vi "Add if Valid.vi"(10 "element":cluster{"Heat":i32, "Prev Steps":T1[]}, 11 "set in":set{cluster{"Heat":i32, "Prev Steps":T1[]}}(c389)) -> (3 "set out":set{cluster{"Heat":i32, "Prev Steps":T1[]}}(c389))   [LabVIEW 2021, in "Heat Map.lvclass"]
uses:
  Heat Map.lvclass
  Direction.ctl
  Heat Map.lvclass/Heat Map.ctl
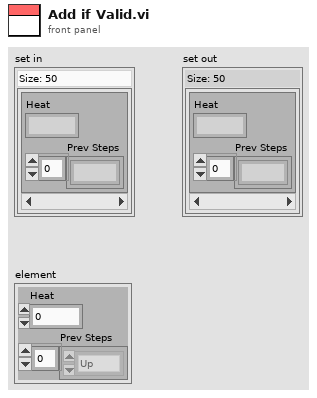
[diagram p1: front panel]
types:
  T1 = typedef "Heat Map.lvclass/Direction.ctl" = enum16{"Up", "Down", "Right", "Left"}
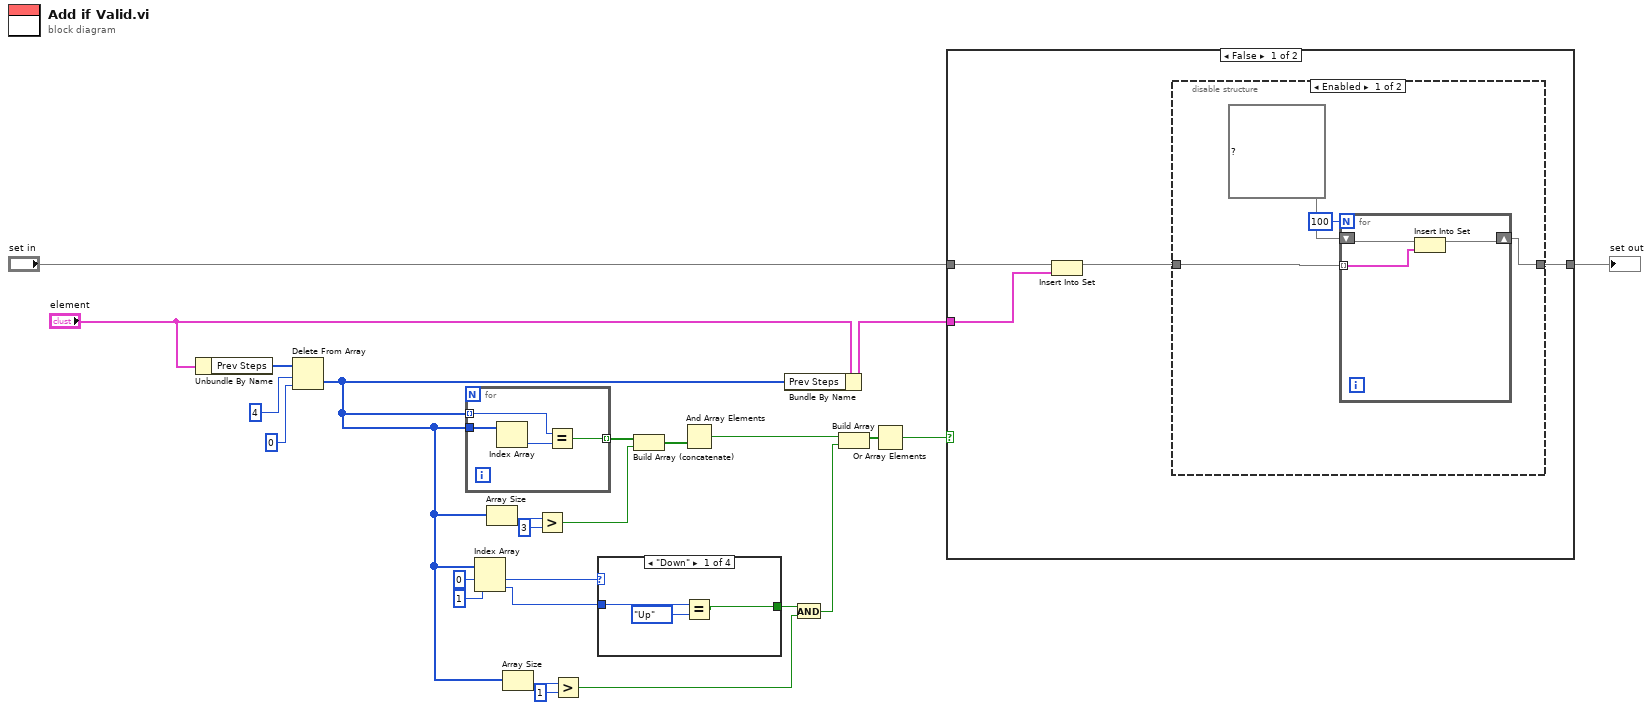
[diagram p0: block diagram]
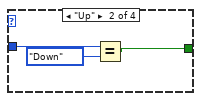
[diagram p4: hidden frame]
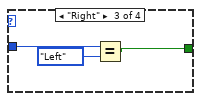
[diagram p5: hidden frame]
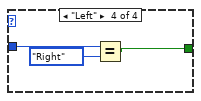
[diagram p6: hidden frame]
diagram:
  n1 = Unbundle By Name("element") -> ("Prev Steps"=w7:T1[])
  n2 = Delete From Array(array=w7, length=4, index=0) -> (deleted portion=w2:T1[])  [unwired: 1 out]
  n3 = for {
    tunnel: w2 -> [w27] mode=indexing
    tunnel: w2 -> [w29]
    tunnel: [w26] -> w23 mode=indexing
    n4 = Index Array(array=w29) -> (element=w28:T1)  [unwired: 1 in]
    n5 = Equal?(x=w27, y=w28) -> (x = y?=w26:bool)
  }
  n6 = Index Array(array=w2, index #1=0 ("index"), index #2=1 ("index")) -> (element #1=w20:T1, element #2=w19:T1)
  n7 = Array Size(array=w2) -> (size(s)=w13:i32)
  n8 = Array Size(array=w2) -> (size(s)=w8:i32)
  n9 = Greater?(x=w13, y=3) -> (0:w11:bool)
  n10 = Greater?(x=w8, y=1) -> (0:w5:bool)
  n11 = case shown="\"Down\"" w20 {
    tunnel: w19 -> [w32 w35 w38 w41]
    tunnel: [w30 w33 w36 w39] -> w17
    frame "Down" {
      n12 = Equal?(x=w32, y=Direction."Up") -> (x = y?=w30:bool)
    }
    frame "Up" {
      n13 = Equal?(x=w35, y=Direction."Down") -> (x = y?=w33:bool)
    }
    frame "Right" {
      n14 = Equal?(x=w38, y=Direction."Left") -> (x = y?=w36:bool)
    }
    frame "Left" {
      n15 = Equal?(x=w41, y=Direction."Right") -> (x = y?=w39:bool)
    }
  }
  n16 = Build Array (concatenate)(w23, w11) -> (w14:bool[])
  n17 = And Array Elements(Boolean array=w14) -> (logical AND=w18:bool)
  n18 = Bundle By Name(cluster="element", "Prev Steps"=w2) -> (w10:cluster{"Heat":i32, "Prev Steps":T1[]})
  n19 = And(x=w17, y=w5) -> (x .and. y?=w6:bool)
  n20 = Build Array(w18, w6) -> (w16:bool[])
  n21 = Or Array Elements(Boolean array=w16) -> (logical OR=w15:bool)
  n22 = case shown="False" w15 {
    tunnel: "set in" -> [w45 w54]
    tunnel: w10 -> [w44 _]
    tunnel: [w42 w54] -> w1
    frame False {
      n23 = Insert Into Set(10:w44, 11:w45) -> (3:w43:set{cluster{"Heat":i32, "Prev Steps":T1[]}})  [unwired: 1 out]
      n24 = disable-structure shown="Enabled" {
        disable-tunnel: w43 -> [w49 w53]
        disable-tunnel: [w47 w53] -> w42
        frame Enabled {
          n25 = for {
            N: 100 -> [_]
            tunnel: w49 -> [w51] mode=indexing
            shift-right: [w50] -> w47
            shift-left: set{cluster{"Heat":i32, "Prev Steps":T1[]}} {} ("set out") -> [w52]
            n26 = Insert Into Set(10:w51, 11:w52) -> (3:w50:set{cluster{"Heat":i32, "Prev Steps":T1[]}})  [unwired: 1 out]
          }
        }
        frame Disabled {
        }
      }
    }
    frame True {
    }
  }
  "set out" <- w1
